vi "rsscope_core_global.vi"() -> ()   [LabVIEW 2014] (continued)
Models"="", "Instrument Options"="", "Flags"=0, "Help"="Sets the timeout between packets in a UART data stream. A new packet starts with the first start bit after the timeout.\n\nAvailable Repeated Capabilities:\nSerialBus: SB1, SB2, SB3, SB4\r\n\nRemote-control command(s):\nBUS<m>:UART:TOUT"}, {"Level"=3, "Class Only"=FALSE, "Identifier"="RSSCOPE_ATTR_PROTOCOL_UART_END_OF_FRAME", "Descriptive Name"="Protocol UART End Of Frame", "Data Type"=0, "Command"="BUS{SerialBus}:UART:EWOR", "Access"=2, "Range Table"="", "Read Callback"="", "Write Callback"="", "Supported Models"="", "Instrument Options"="", "Flags"=0, "Help"="Sets the end pattern of the packets. A new packet starts with the first start bit after the defined end pattern. This property using hexadecimal format (prefix #H).\n\nAvailable Repeated Capabilities:\nSerialBus: SB1, SB2, SB3, SB4\r\n\nRemote-control command(s):\nBUS<m>:UART:EWORd"}, {"Level"=3, "Class Only"=TRUE, "Identifier"="", "Descriptive Name"="RX", "Data Type"=0, "Command"="", "Access"=0, "Range Table"="", "Read Callback"="", "Write Callback"="", "Supported Models"="", "Instrument Options"="", "Flags"=0, "Help"="Configures UART RX properties."}, {"Level"=4, "Class Only"=FALSE, "Identifier"="RSSCOPE_ATTR_PROTOCOL_UART_RX_SOURCE", "Descriptive Name"="Protocol UART RX Source", "Data Type"=0, "Command"="BUS{SerialBus}:UART:RX:SOUR", "Access"=2, "Range Table"="rsscope_rngProtocolWaveformSource", "Read Callback"="", "Write Callback"="", "Supported Models"="", "Instrument Options"="", "Flags"=0, "Help"="Selects the input channel for the receiver signal.\n\nAvailable Repeated Capabilities:\nSerialBus: SB1, SB2, SB3, SB4\r\n\nRemote-control command(s):\nBUS<m>:UART:RX:SOURce"}, {"Level"=4, "Class Only"=FALSE, "Identifier"="RSSCOPE_ATTR_PROTOCOL_UART_RX_THRESHOLD", "Descriptive Name"="Protocol UART RX Threshold", "Data Type"=1, "Command"="BUS{SerialBus}:UART:RX:THR", "Access"=2, "Range Table"="rsscope_rngProtocolThresholdUART", "Read Callback"="", "Write Callback"="", "Supported Models"="", "Instrument Options"="", "Flags"=0, "Help"="Sets a user-defined threshold value for the Rx line.\n\nAvailable Repeated Capabilities:\nSerialBus: SB1, SB2, SB3, SB4\r\n\nRemote-control command(s):\nBUS<m>:UART:RX:THReshold"}, {"Level"=3, "Class Only"=TRUE, "Identifier"="", "Descriptive Name"="TX", "Data Type"=0, "Command"="", "Access"=0, "Range Table"="", "Read Callback"="", "Write Callback"="", "Supported Models"="", "Instrument Options"="", "Flags"=0, "Help"="Configures UART TX properties."}, {"Level"=4, "Class Only"=FALSE, "Identifier"="RSSCOPE_ATTR_PROTOCOL_UART_TX_SOURCE", "Descriptive Name"="Protocol UART TX Source", "Data Type"=0, "Command"="BUS{SerialBus}:UART:TX:SOUR", "Access"=2, "Range Table"="rsscope_rngProtocolWaveformSource", "Read Callback"="", "Write Callback"="", "Supported Models"="", "Instrument Options"="", "Flags"=0, "Help"="Selects the input channel for the transmitter signal.\n\nAvailable Repeated Capabilities:\nSerialBus: SB1, SB2, SB3, SB4\r\n\nRemote-control command(s):\nBUS<m>:UART:TX:SOURce"}, {"Level"=4, "Class Only"=FALSE, "Identifier"="RSSCOPE_ATTR_PROTOCOL_UART_TX_THRESHOLD", "Descriptive Name"="Protocol UART TX Threshold", "Data Type"=1, "Command"="BUS{SerialBus}:UART:TX:THR", "Access"=2, "Range Table"="rsscope_rngProtocolThresholdUART", "Read Callback"="", "Write Callback"="", "Supported Models"="", "Instrument Options"="", "Flags"=0, "Help"="Sets a user-defined threshold value for the Tx line.\n\nAvailable Repeated Capabilities:\nSerialBus: SB1, SB2, SB3, SB4\r\n\nRemote-control command(s):\nBUS<m>:UART:TX:THReshold"}, {"Level"=2, "Class Only"=TRUE, "Identifier"="", "Descriptive Name"="LIN", "Data Type"=0, "Command"="", "Access"=0, "Range Table"="", "Read Callback"="", "Write Callback"="", "Supported Models"="", "Instrument Options"="", "Flags"=0, "Help"="This class contains attributes that configure the LIN (Local Interconnect Network)\n\nAttributes in this class require option R&S RTO-K3."}, {"Level"=3, "Class Only"=FALSE, "Identifier"="RSSCOPE_ATTR_PROTOCOL_LIN_SOURCE", "Descriptive Name"="Protocol LIN Source", "Data Type"=0, "Command"="BUS{SerialBus}:LIN:DATA:SOUR", "Access"=2, "Range Table"="rsscope_rngProtocolWaveformSource", "Read Callback"="", "Write Callback"="", "Supported Models"="", "Instrument Options"="K0|K3", "Flags"=0, "Help"="Selects source waveform of the data line.\n\nAvailable Repeated Capabilities:\nSerialBus: SB1, SB2, SB3, SB4\r\n\nRemote-control command(s):\nBUS<m>:LIN:DATA:SOURce"}, {"Level"=3, "Class Only"=FALSE, "Identifier"="RSSCOPE_ATTR_PROTOCOL_LIN_THRESHOLD", "Descriptive Name"="Protocol LIN Threshold", "Data Type"=1, "Command"="BUS{SerialBus}:LIN:DATA:THR", "Access"=2, "Range Table"="rsscope_rngProtocolThreshold", "Read Callback"="", "Write Callback"="", "Supported Models"="", "Instrument Options"="K0|K3", "Flags"=0, "Help"="Sets threshold value for digitization of analog signals.\n\nAlternatively, you can set the threshold according to the signal technology with RSSCOPE_ATTR_PROTOCOL_LIN_TECHNOLOGY\n\nAvailable Repeated Capabilities:\nSerialBus: SB1, SB2, SB3, SB4\r\n\nRemote-control command(s):\nBUS<m>:LIN:DATA:THReshold"}, {"Level"=3, "Class Only"=FALSE, "Identifier"="RSSCOPE_ATTR_PROTOCOL_LIN_TECHNOLOGY", "Descriptive Name"="Protocol LIN Technology", "Data Type"=0, "Command"="BUS{SerialBus}:LIN:TECH", "Access"=2, "Range Table"="rsscope_rngProtocolLINTechnology", "Read Callback"="", "Write Callback"="", "Supported Models"="", "Instrument Options"="K0|K3", "Flags"=0, "Help"="Selecs the threshold voltage for various signal technologies from a list.\n\nFor user defined values set to manual and use RSSCOPE_ATTR_PROTOCOL_LIN_THRESHOLD.\n\nAvailable Repeated Capabilities:\nSerialBus: SB1, SB2, SB3, SB4\r\n\nRemote-control command(s):\nBUS<m>:LIN:TECHnology"}, {"Level"=3, "Class Only"=FALSE, "Identifier"="RSSCOPE_ATTR_PROTOCOL_LIN_STANDARD", "Descriptive Name"="Protocol LIN Standard", "Data Type"=0, "Command"="BUS{SerialBus}:LIN:STAN", "Access"=2, "Range Table"="rsscope_rngProtocolLINStandard", "Read Callback"="", "Write Callback"="", "Supported Models"="", "Instrument Options"="K0|K3", "Flags"=0, "Help"="This attribute selects the version of the LIN standard.\n\nAvailable Repeated Capabilities:\nSerialBus: SB1, SB2, SB3, SB4\r\n\nRemote-control command(s):\nBUS<m>:LIN:STANdard"}, {"Level"=3, "Class Only"=FALSE, "Identifier"="RSSCOPE_ATTR_PROTOCOL_LIN_BIT_RATE", "Descriptive Name"="Protocol LIN Bit Rate", "Data Type"=0, "Command"="BUS{SerialBus}:LIN:BITR", "Access"=2, "Range Table"="rsscope_rngProtocolLINBitRate", "Read Callback"="", "Write Callback"="", "Supported Models"="", "Instrument Options"="K0|K3", "Flags"=0, "Help"="Sets the number of transmitted bits per second.\n\nNote(s):\n(1) For LIN standard &apos;J2602&apos;, the bit rate is 10417 kbit/s and cannot be changed.\n\nAvailable Repeated Capabilities:\nSerialBus: SB1, SB2, SB3, SB4\r\n\nRemote-control command(s):\nBUS<m>:LIN:BITRate"}, {"Level"=3, "Class Only"=FALSE, "Identifier"="RSSCOPE_ATTR_PROTOCOL_LIN_POLARITY", "Descriptive Name"="Protocol LIN Polarity", "Data Type"=0, "Command"="BUS{SerialBus}:LIN:POL", "Access"=2, "Range Table"="rsscope_rngProtocolPolarity", "Read Callback"="", "Write Callback"="", "Supported Models"="", "Instrument Options"="K0|K3", "Flags"=0, "Help"="Sets the idle state of the bus. The idle state is the rezessive state and corresponds to a logic 1.\n\nAvailable Repeated Capabilities:\nSerialBus: SB1, SB2, SB3, SB4\r\n\nRemote-control command(s):\nBUS<m>:LIN:POLarity"}, {"Level"=3, "Class Only"=FALSE, "Identifier"="RSSCOPE_ATTR_PROTOCOL_LIN_SELECTED_FRAME", "Descriptive Name"="Protocol LIN Selected Frame", "Data Type"=0, "Command"="", "Access"=2, "Range Table"="", "Read Callback"="", "Write Callback"="", "Supported Models"="", "Instrument Options"="", "Flags"=0, "Help"="Sets selector repeated capability Frame.\n\nAvailable Repeated Capabilities:\nNone\n\nRemote-control command(s):\ncmd"}, {"Level"=3, "Class Only"=FALSE, "Identifier"="RSSCOPE_ATTR_PROTOCOL_LIN_FRAME_COUNT", "Descriptive Name"="Protocol LIN Frame Count", "Data Type"=0, "Command"="BUS{SerialBus}:LIN:FCO?", "Access"=0, "Range Table"="", "Read Callback"="", "Write Callback"="", "Supported Models"="", "Instrument Options"="K0|K3", "Flags"=0, "Help"="Returns number of decoded frames.\n\nAvailable Repeated Capabilities:\nSerialBus: SB1, SB2, SB3, SB4\r\n\nRemote-control command(s):\nBUS<m>:LIN:FCOunt?"}, {"Level"=3, "Class Only"=FALSE, "Identifier"="RSSCOPE_ATTR_PROTOCOL_LIN_FRAME_STATUS", "Descriptive Name"="Protocol LIN Frame Status", "Data Type"=0, "Command"="BUS{SerialBus}:LIN:FRAM<Frame>:STAT?", "Access"=0, "Range Table"="RsScope_rngLINFrameStatus", "Read Callback"="rsscope_FormatLINFrameRepCapInt32_ReadCallback.vi", "Write Callback"="", "Supported Models"="", "Instrument Options"="K3", "Flags"=0, "Help"="The overall state of the frame.\n\nAvailable Repeated Capabilities:\nSerialBus: SB1, SB2, SB3, SB4\r\n\nRemote-control command(s):\nBUS<m>:LIN:FRAMe<n>:STATus?"}, {"Level"=3, "Class Only"=FALSE, "Identifier"="RSSCOPE_ATTR_PROTOCOL_LIN_FRAME_START", "Descriptive Name"="Protocol LIN Frame Start", "Data Type"=1, "Command"="BUS{SerialBus}:LIN:FRAM<Frame>:STAR?", "Access"=0, "Range Table"="", "Read Callback"="rsscope_FormatLINFrameRepCapReal64_ReadCallback.vi", "Write Callback"="", "Supported Models"="", "Instrument Options"="K3", "Flags"=0, "Help"="Return the start time of the selected frame.\n\nAvailable Repeated Capabilities:\nSerialBus: SB1, SB2, SB3, SB4\r\n\nRemote-control command(s):\nBUS<m>:LIN:FRAMe<n>:STARt?"}, {"Level"=3, "Class Only"=FALSE, "Identifier"="RSSCOPE_ATTR_PROTOCOL_LIN_FRAME_STOP", "Descriptive Name"="Protocol LIN Frame Stop", "Data Type"=1, "Command"="BUS{SerialBus}:LIN:FRAM<Frame>:STOP?", "Access"=0, "Range Table"="", "Read Callback"="rsscope_FormatLINFrameRepCapReal64_ReadCallback.vi", "Write Callback"="", "Supported Models"="", "Instrument Options"="K3", "Flags"=0, "Help"="Return the stop time of the selected frame.\n\nAvailable Repeated Capabilities:\nSerialBus: SB1, SB2, SB3, SB4\r\n\nRemote-control command(s):\nBUS<m>:LIN:FRAMe<n>:STOP?"}, {"Level"=3, "Class Only"=FALSE, "Identifier"="RSSCOPE_ATTR_PROTOCOL_LIN_FRAME_VERSION", "Descriptive Name"="Protocol LIN Frame Version", "Data Type"=0, "Command"="BUS{SerialBus}:LIN:FRAM<Frame>:VERS?", "Access"=0, "Range Table"="RsScope_rngLINFrameVersion", "Read Callback"="rsscope_FormatLINFrameRepCapInt32_ReadCallback.vi", "Write Callback"="", "Supported Models"="", "Instrument Options"="K3", "Flags"=0, "Help"="Returns the version of the LIN standard for the specified frame.\n\nAvailable Repeated Capabilities:\nSerialBus: SB1, SB2, SB3, SB4\r\n\nRemote-control command(s):\nBUS<m>:LIN:FRAMe<n>:VERSion?"}, {"Level"=3, "Class Only"=FALSE, "Identifier"="RSSCOPE_ATTR_PROTOCOL_LIN_FRAME_ID_VALUE", "Descriptive Name"="Protocol LIN Frame ID Value", "Data Type"=0, "Command"="BUS{SerialBus}:LIN:FRAM<Frame>:IDV?", "Access"=0, "Range Table"="", "Read Callback"="rsscope_FormatLINFrameRepCapInt32_ReadCallback.vi", "Write Callback"="", "Supported Models"="", "Instrument Options"="K3", "Flags"=0, "Help"="Returns the version of the LIN standard for the specified frame.\n\nAvailable Repeated Capabilities:\nSerialBus: SB1, SB2, SB3, SB4\r\n\nRemote-control command(s):\nBUS<m>:LIN:FRAMe<n>:IDValue?"}, {"Level"=3, "Class Only"=FALSE, "Identifier"="RSSCOPE_ATTR_PROTOCOL_LIN_FRAME_ID_PARITY", "Descriptive Name"="Protocol LIN Frame ID Parity", "Data Type"=0, "Command"="BUS{SerialBus}:LIN:FRAM<Frame>:IDPV?", "Access"=0, "Range Table"="", "Read Callback"="rsscope_FormatLINFrameRepCapInt32_ReadCallback.vi", "Write Callback"="", "Supported Models"="", "Instrument Options"="K3", "Flags"=0, "Help"="Returns the value of the identifier parity bits of the selected frame.\n\nAvailable Repeated Capabilities:\nSerialBus: SB1, SB2, SB3, SB4\r\n\nRemote-control command(s):\nBUS<m>:LIN:FRAMe<n>:IDPValue?"}, {"Level"=3, "Class Only"=FALSE, "Identifier"="RSSCOPE_ATTR_PROTOCOL_LIN_FRAME_ID_STATUS", "Descriptive Name"="Protocol LIN Frame ID Status", "Data Type"=0, "Command"="BUS{SerialBus}:LIN:FRAM<Frame>:IDST?", "Access"=0, "Range Table"="RsScope_rngLINFieldStatus", "Read Callback"="rsscope_FormatLINFrameRepCapInt32_ReadCallback.vi", "Write Callback"="", "Supported Models"="", "Instrument Options"="K3", "Flags"=0, "Help"="Returns the identifier state of the selected frame.\n\nAvailable Repeated Capabilities:\nSerialBus: SB1, SB2, SB3, SB4\r\n\nRemote-control command(s):\nBUS<m>:LIN:FRAMe<n>:IDSTate?"}, {"Level"=3, "Class Only"=FALSE, "Identifier"="RSSCOPE_ATTR_PROTOCOL_LIN_FRAME_SYNC_STATUS", "Descriptive Name"="Protocol LIN Frame Sync Status", "Data Type"=0, "Command"="BUS{SerialBus}:LIN:FRAM<Frame>:SYST?", "Access"=0, "Range Table"="RsScope_rngLINFieldStatus", "Read Callback"="rsscope_FormatLINFrameRepCapInt32_ReadCallback.vi", "Write Callback"="", "Supported Models"="", "Instrument Options"="K3", "Flags"=0, "Help"="Returns the state of the sync field for the specified frame.\n\nAvailable Repeated Capabilities:\nSerialBus: SB1, SB2, SB3, SB4\r\n\nRemote-control command(s):\nBUS<m>:LIN:FRAMe<n>:SYSTate?"}, {"Level"=3, "Class Only"=FALSE, "Identifier"="RSSCOPE_ATTR_PROTOCOL_LIN_FRAME_CHECKSUM_STATUS", "Descriptive Name"="Protocol LIN Frame Checksum Status", "Data Type"=0, "Command"="BUS{SerialBus}:LIN:FRAM<Frame>:CSST?", "Access"=0, "Range Table"="RsScope_rngLINFieldStatus", "Read Callback"="rsscope_FormatLINFrameRepCapInt32_ReadCallback.vi", "Write Callback"="", "Supported Models"="", "Instrument Options"="K3", "Flags"=0, "Help"="Returns the checksum state of the specified frame.\n\nAvailable Repeated Capabilities:\nSerialBus: SB1, SB2, SB3, SB4\r\n\nRemote-control command(s):\nBUS<m>:LIN:FRAMe<n>:CSSTate?"}, {"Level"=3, "Class Only"=FALSE, "Identifier"="RSSCOPE_ATTR_PROTOCOL_LIN_FRAME_CHECKSUM_VALUE", "Descriptive Name"="Protocol LIN Frame Checksum Value", "Data Type"=0, "Command"="BUS{SerialBus}:LIN:FRAM<Frame>:CSV?", "Access"=0, "Range Table"="", "Read Callback"="rsscope_FormatLINFrameRepCapInt32_ReadCallback.vi", "Write Callback"="", "Supported Models"="", "Instrument Options"="K3", "Flags"=0, "Help"="Returns the checksum value of the specified frame.\n\nAvailable Repeated Capabilities:\nSerialBus: SB1, SB2, SB3, SB4\r\n\nRemote-control command(s):\nBUS<m>:LIN:FRAMe<n>:CSValue?"}, {"Level"=3, "Class Only"=FALSE, "Identifier"="RSSCOPE_ATTR_PROTOCOL_LIN_FRAME_BIT_RATE", "Descriptive Name"="Protocol LIN Frame Bit Rate", "Data Type"=5, "Command"="BUS{SerialBus}:LIN:FRAM<Frame>:BITR?", "Access"=0, "Range Table"="", "Read Callback"="rsscope_FormatLINFrameRepCapInt64_ReadCallback.vi", "Write Callback"="", "Supported Models"="", "Instrument Options"="K3", "Flags"=0, "Help"="Returns the primary bit rate.\n\nAvailable Repeated Capabilities:\nSerialBus: SB1, SB2, SB3, SB4\r\n\nRemote-control command(s):\nBUS<m>:LIN:FRAMe<n>:BITRate?"}, {"Level"=3, "Class Only"=FALSE, "Identifier"="RSSCOPE_ATTR_PROTOCOL_LIN_FRAME_LABEL", "Descriptive Name"="Protocol LIN Frame Label", "Data Type"=2, "Command"="BUS{SerialBus}:LIN:FRAM<Frame>:SYMB?", "Access"=0, "Range Table"="", "Read Callback"="rsscope_FormatLINFrameRepCapString_ReadCallback.vi", "Write Callback"="", "Supported Models"="", "Instrument Options"="K3", "Flags"=0, "Help"="This attribute returns the symbolic label of the specified frame if the label list is enabled.\n\nAvailable Repeated Capabilities:\nSerialBus: SB1, SB2, SB3, SB4\r\n\nRemote-control command(s):\nBUS<m>:LIN:FRAMe<n>:SYMBol?"}, {"Level"=3, "Class Only"=FALSE, "Identifier"="RSSCOPE_ATTR_PROTOCOL_LIN_SELECTED_BYTE", "Descriptive Name"="Protocol LIN Selected Byte", "Data Type"=0, "Command"="", "Access"=2, "Range Table"="", "Read Callback"="", "Write Callback"="", "Supported Models"="", "Instrument Options"="", "Flags"=0, "Help"="Sets selector repeated capability Byte.\n\nAvailable Repeated Capabilities:\nNone\n\nRemote-control command(s):\ncmd"}, {"Level"=3, "Class Only"=FALSE, "Identifier"="RSSCOPE_ATTR_PROTOCOL_LIN_FRAME_BYTE_DATA", "Descriptive Name"="Protocol LIN Frame Byte Data", "Data Type"=0, "Command"="BUS{SerialBus}:LIN:FRAM<Frame>:BYTE<Byte>:VAL?", "Access"=0, "Range Table"="", "Read Callback"="rsscope_FormatLINByteRepCapInt32_ReadCallback.vi", "Write Callback"="", "Supported Models"="", "Instrument Options"="K3", "Flags"=0, "Help"="Value of the specified byte.\n\nAvailable Repeated Capabilities:\nSerialBus: SB1, SB2, SB3, SB4\r\n\nRemote-control command(s):\nBUS<m>:LIN:FRAMe<n>:BYTE<o>:VALue?"}, {"Level"=3, "Class Only"=FALSE, "Identifier"="RSSCOPE_ATTR_PROTOCOL_LIN_FRAME_BYTE_STATUS", "Descriptive Name"="Protocol LIN Frame Byte Status", "Data Type"=0, "Command"="BUS{SerialBus}:LIN:FRAM<Frame>:BYTE<Byte>:STAT?", "Access"=0, "Range Table"="RsScope_rngLINFieldStatus", "Read Callback"="rsscope_FormatLINByteRepCapInt32_ReadCallback.vi", "Write Callback"="", "Supported Models"="", "Instrument Options"="K3", "Flags"=0, "Help"="Returns the data state for the specified frame.\n\nAvailable Repeated Capabilities:\nSerialBus: SB1, SB2, SB3, SB4\r\n\nRemote-control command(s):\nBUS<m>:LIN:FRAMe<n>:BYTE<o>:STATe?"}, {"Level"=2, "Class Only"=TRUE, "Identifier"="", "Descriptive Name"="CAN", "Data Type"=0, "Command"="", "Access"=0, "Range Table"="", "Read Callback"="", "Write Callback"="", "Supported Models"="", "Instrument Options"="", "Flags"=0, "Help"="This class contains attributes that configure the CAN (Controller Area Network)\n\nAttributes in this class require option R&S RTO-K3."}, {"Level"=3, "Class Only"=FALSE, "Identifier"="RSSCOPE_ATTR_PROTOCOL_CAN_SOURCE", "Descriptive Name"="Protocol CAN Source", "Data Type"=0, "Command"="BUS{SerialBus}:CAN:DATA:SOUR", "Access"=2, "Range Table"="rsscope_rngProtocolWaveformSource", "Read Callback"="", "Write Callback"="", "Supported Models"="", "Instrument Options"="K0|K3", "Flags"=0, "Help"="Selects source waveform of the data line.\n\nAvailable Repeated Capabilities:\nSerialBus: SB1, SB2, SB3, SB4\r\n\nRemote-control command(s):\nBUS<m>:CAN:DATA:SOURce"}, {"Level"=3, "Class Only"=FALSE, "Identifier"="RSSCOPE_ATTR_PROTOCOL_CAN_LINE_TYPE", "Descriptive Name"="Protocol CAN Line Type", "Data Type"=0, "Command"="BUS{SerialBus}:CAN:TYPE", "Access"=2, "Range Table"="rsscope_rngProtocolCANLineType", "Read Callback"="", "Write Callback"="", "Supported Models"="", "Instrument Options"="K0|K3", "Flags"=0, "Help"="Selects the CAN-High or CAN-Low line. Both lines are required for differential signal transmission used by CAN.\n\nAvailable Repeated Capabilities:\nSerialBus: SB1, SB2, SB3, SB4\r\n\nRemote-control command(s):\nBUS<m>:CAN:TYPE"}, {"Level"=3, "Class Only"=FALSE, "Identifier"="RSSCOPE_ATTR_PROTOCOL_CAN_THRESHOLD", "Descriptive Name"="Protocol CAN Threshold", "Data Type"=1, "Command"="BUS{SerialBus}:CAN:DATA:THR", "Access"=2, "Range Table"="rsscope_rngProtocolThreshold", "Read Callback"="", "Write Callback"="", "Supported Models"="", "Instrument Options"="K0|K3", "Flags"=0, "Help"="Sets threshold value for digitization of analog signals.\n\nAlternatively, you can set the threshold according to the signal technology with RSSCOPE_ATTR_PROTOCOL_CAN_TECHNOLOGY\n\nAvailable Repeated Capabilities:\nSerialBus: SB1, SB2, SB3, SB4\r\n\nRemote-control command(s):\nBUS<m>:CAN:DATA:THReshold"}, {"Level"=3, "Class Only"=FALSE, "Identifier"="RSSCOPE_ATTR_PROTOCOL_CAN_TECHNOLOGY", "Descriptive Name"="Protocol CAN Technology", "Data Type"=0, "Command"="BUS{SerialBus}:CAN:TECH", "Access"=2, "Range Table"="rsscope_rngProtocolCANTechnology", "Read Callback"="", "Write Callback"="", "Supported Models"="", "Instrument Options"="K0|K3", "Flags"=0, "Help"="Selecs the threshold voltage for various signal technologies from a list.\n\nFor user defined values set to manual and use RSSCOPE_ATTR_PROTOCOL_LIN_THRESHOLD.\n\nAvailable Repeated Capabilities:\nSerialBus: SB1, SB2, SB3, SB4\r\n\nRemote-control command(s):\nBUS<m>:CAN:TECHnology"}, {"Level"=3, "Class Only"=FALSE, "Identifier"="RSSCOPE_ATTR_PROTOCOL_CAN_BIT_RATE", "Descriptive Name"="Protocol CAN Bit Rate", "Data Type"=0, "Command"="BUS{SerialBus}:CAN:BITR", "Access"=2, "Range Table"="rsscope_rngProtocolCANBitRate", "Read Callback"="", "Write Callback"="", "Supported Models"="", "Instrument Options"="K0|K3", "Flags"=0, "Help"="Sets the number of transmitted bits per second.\n\nAvailable Repeated Capabilities:\nSerialBus: SB1, SB2, SB3, SB4\r\n\nRemote-control command(s):\nBUS<m>:CAN:BITRate"}, {"Level"=3, "Class Only"=FALSE, "Identifier"="RSSCOPE_ATTR_PROTOCOL_CAN_FD_ENABLED", "Descriptive Name"="Protocol CAN FD Enabled", "Data Type"=3, "Command"="BUS{SerialBus}:CAN:FDAT:ENAB", "Access"=2, "Range Table"="", "Read Callback"="", "Write Callback"="", "Supported Models"="", "Instrument Options"="K9", "Flags"=0, "Help"="Enables the CAN FD protocol configuration.\n\nAvailable Repeated Capabilities:\nSerialBus: SB1, SB2, SB3, SB4\r\n\nRemote-control command(s):\nBUS<m>:CAN:FDATa:ENABle"}, {"Level"=3, "Class Only"=FALSE, "Identifier"="RSSCOPE_ATTR_PROTOCOL_CAN_FD_BIT_RATE", "Descriptive Name"="Protocol CAN FD Bit Rate", "Data Type"=0, "Command"="BUS{SerialBus}:CAN:FDAT:DBIT", "Access"=2, "Range Table"="rsscope_rngProtocolCANFDBitRate", "Read Callback"="", "Write Callback"="", "Supported Models"="", "Instrument Options"="K9", "Flags"=0, "Help"="Sets the bit rate of the data phase. The data rate can be higher than the arbitration rate, but it is uniform and fixed for a given CAN FD bus.\n\nAvailable Repeated Capabilities:\nSerialBus: SB1, SB2, SB3, SB4\r\n\nRemote-control command(s):\nBUS<m>:CAN:FDATa:DBITrate"}, {"Level"=3, "Class Only"=FALSE, "Identifier"="RSSCOPE_ATTR_PROTOCOL_CAN_JUMP_WIDTH", "Descriptive Name"="Protocol CAN Jump Width", "Data Type"=1, "Command"="BUS{SerialBus}:CAN:JWID", "Access"=2, "Range Table"="rsscope_rngProtocolCANJumpWidth", "Read Callback"="", "Write Callback"="", "Supported Models"="", "Instrument Options"="K0|K3", "Flags"=0, "Help"="This attribute configures maximum number of time quanta for phase correction. This mean Time segment1 may be lengthened or Time segment2 may be shortened due to resynchronization.\n\nAvailable Repeated Capabilities:\nSerialBus: SB1, SB2, SB3, SB4\r\n\nRemote-control command(s):\nBUS<m>:CAN:JWIDth"}, {"Level"=3, "Class Only"=FALSE, "Identifier"="RSSCOPE_ATTR_PROTOCOL_CAN_SAMPLE_POINT_REL", "Descriptive Name"="Protocol CAN Sample Point Rel", "Data Type"=1, "Command"="BUS{SerialBus}:CAN:SAMP", "Access"=2, "Range Table"="rsscope_rngProtocolCANSamplePoint", "Read Callback"="", "Write Callback"="", "Supported Models"="", "Instrument Options"="K0|K3", "Flags"=0, "Help"="Sets the position of the sample point within the bit in percent ot the nominal bit time.\n\nAvailable Repeated Capabilities:\nSerialBus: SB1, SB2, SB3, SB4\r\n\nRemote-control command(s):\nBUS<m>:CAN:SAMPlepoint"}, {"Level"=3, "Class Only"=FALSE, "Identifier"="RSSCOPE_ATTR_PROTOCOL_CAN_FD_JUMP_WIDTH", "Descriptive Name"="Protocol CAN FD Jump Width", "Data Type"=1, "Command"="BUS{SerialBus}:CAN:FDAT:JWID", "Access"=2, "Range Table"="rsscope_rngProtocolCANJumpWidth", "Read Callback"="", "Write Callback"="", "Supported Models"="", "Instrument Options"="K0|K3", "Flags"=0, "Help"="This attribute configures maximum number of time quanta for phase correction. This mean Time segment1 may be lengthened or Time segment2 may be shortened due to resynchronization.\n\nAvailable Repeated Capabilities:\nSerialBus: SB1, SB2, SB3, SB4\r\n\nRemote-control command(s):\nBUS<m>:CAN:FDATa:JWIDth"}, {"Level"=3, "Class Only"=FALSE, "Identifier"="RSSCOPE_ATTR_PROTOCOL_CAN_FD_SAMPLE_POINT_REL", "Descriptive Name"="Protocol CAN FD Sample Point Rel", "Data Type"=1, "Command"="BUS{SerialBus}:CAN:FDAT:SAMP", "Access"=2, "Range Table"="rsscope_rngProtocolCANSamplePoint", "Read Callback"="", "Write Callback"="", "Supported Models"="", "Instrument Options"="K0|K3", "Flags"=0, "Help"="Sets the position of the sample point within the bit in percent ot the nominal bit time.\n\nAvailable Repeated Capabilities:\nSerialBus: SB1, SB2, SB3, SB4\r\n\nRemote-control command(s):\nBUS<m>:CAN:FDATa:SAMPlepoint"}, {"Level"=3, "Class Only"=FALSE, "Identifier"="RSSCOPE_ATTR_PROTOCOL_CAN_FD_STANDARD", "Descriptive Name"="Protocol CAN FD Standard", "Data Type"=0, "Command"="BUS{SerialBus}:CAN:FDAT:PST", "Access"=2, "Range Table"="RsScope_rngCANFDStandard", "Read Callback"="", "Write Callback"="", "Supported Models"="", "Instrument Options"="K3", "Flags"=0, "Help"="Only available for CAN FD buses. Selects whether the tested signal is an ISO CAN FD signal or not.\n\nAvailable Repeated Capabilities:\nSerialBus: SB1, SB2, SB3, SB4\r\n\nRemote-control command(s):\nBUS<m>:CAN:FDATa:PSTandard"}, {"Level"=3, "Class Only"=FALSE, "Identifier"="RSSCOPE_ATTR_PROTOCOL_CAN_SELECTED_FRAME", "Descriptive Name"="Protocol CAN Selected Frame", "Data Type"=0, "Command"="", "Access"=2, "Range Table"="", "Read Callback"="", "Write Callback"="", "Supported Models"="", "Instrument Options"="", "Flags"=0, "Help"="Sets selector repeated capability Frame.\n\nAvailable Repeated Capabilities:\nNone\n\nRemote-control command(s):\ncmd"}, {"Level"=3, "Class Only"=FALSE, "Identifier"="RSSCOPE_ATTR_PROTOCOL_CAN_FRAME_COUNT", "Descriptive Name"="Protocol CAN Frame Count", "Data Type"=0, "Command"="BUS{SerialBus}:CAN:FCO?", "Access"=0, "Range Table"="", "Read Callback"="", "Write Callback"="", "Supported Models"="", "Instrument Options"="K0|K3", "Flags"=0, "Help"="Returns number of decoded frames.\n\nAvailable Repeated Capabilities:\nSerialBus: SB1, SB2, SB3, SB4\r\n\nRemote-control command(s):\nBUS<m>:CAN:FCOunt?"}, {"Level"=3, "Class Only"=FALSE, "Identifier"="RSSCOPE_ATTR_PROTOCOL_CAN_FRAME_STANDARD", "Descriptive Name"="Protocol CAN Frame Standard", "Data Type"=0, "Command"="BUS{SerialBus}:CAN:FDAT:FRAM<Frame>:STAN?", "Access"=0, "Range Table"="rsscope_rngCANStandard", "Read Callback"="rsscope_FormatCANFrameRepCapInt32_ReadCallback.vi", "Write Callback"="", "Supported Models"="", "Instrument Options"="K9", "Flags"=0, "Help"="Returns the CAN standard.\n\nAvailable Repeated Capabilities:\nSerialBus: SB1, SB2, SB3, SB4\r\n\nRemote-control command(s):\nBUS<m>:CAN:FDATa:FRAMe<n>:STANdard?"}, {"Level"=3, "Class Only"=FALSE, "Identifier"="RSSCOPE_ATTR_PROTOCOL_CAN_FRAME_STATUS", "Descriptive Name"="Protocol CAN Frame Status", "Data Type"=0, "Command"="BUS{SerialBus}:CAN:FRAM<Frame>:STAT?", "Access"=0, "Range Table"="RsScope_rngCANFrameStatus", "Read Callback"="rsscope_FormatCANFrameRepCapInt32_ReadCallback.vi", "Write Callback"="", "Supported Models"="", "Instrument Options"="K3", "Flags"=0, "Help"="The overall state of the frame.\n\nAvailable Repeated Capabilities:\nSerialBus: SB1, SB2, SB3, SB4\r\n\nRemote-control command(s):\nBUS<m>:CAN:FRAMe<n>:STATus?"}, {"Level"=3, "Class Only"=FALSE, "Identifier"="RSSCOPE_ATTR_PROTOCOL_CAN_FRAME_START", "Descriptive Name"="Protocol CAN Frame Start", "Data Type"=1, "Command"="BUS{SerialBus}:CAN:FRAM<Frame>:STAR?", "Access"=0, "Range Table"="", "Read Callback"="rsscope_FormatCANFrameRepCapReal64_ReadCallback.vi", "Write Callback"="", "Supported Models"="", "Instrument Options"="K3", "Flags"=0, "Help"="Return the start time of the selected frame.\n\nAvailable Repeated Capabilities:\nSerialBus: SB1, SB2, SB3, SB4\r\n\nRemote-control command(s):\nBUS<m>:CAN:FRAMe<n>:STARt?"}, {"Level"=3, "Class Only"=FALSE, "Identifier"="RSSCOPE_ATTR_PROTOCOL_CAN_FRAME_STOP", "Descriptive Name"="Protocol CAN Frame Stop", "Data Type"=1, "Command"="BUS{SerialBus}:CAN:FRAM<Frame>:STOP?", "Access"=0, "Range Table"="", "Read Callback"="rsscope_FormatCANFrameRepCapReal64_ReadCallback.vi", "Write Callback"="", "Supported Models"="", "Instrument Options"="K3", "Flags"=0, "Help"="Return the stop time of the selected frame.\n\nAvailable Repeated Capabilities:\nSerialBus: SB1, SB2, SB3, SB4\r\n\nRemote-control command(s):\nBUS<m>:CAN:FRAMe<n>:STOP?"}, {"Level"=3, "Class Only"=FALSE, "Identifier"="RSSCOPE_ATTR_PROTOCOL_CAN_FRAME_TYPE", "Descriptive Name"="Protocol CAN Frame Type", "Data Type"=0, "Command"="BUS{SerialBus}:CAN:FRAM<Frame>:TYPE?", "Access"=0, "Range Table"="RsScope_rngProtocolCANFrameType", "Read Callback"="rsscope_FormatCANFrameRepCapInt32_ReadCallback.vi", "Write Callback"="", "Supported Models"="", "Instrument Options"="K3", "Flags"=0, "Help"="Returns the frame type of the selected frame.\n\nAvailable Repeated Capabilities:\nSerialBus: SB1, SB2, SB3, SB4\r\n\nRemote-control command(s):\nBUS<m>:CAN:FRAMe<n>:TYPE?"}, {"Level"=3, "Class Only"=FALSE, "Identifier"="RSSCOPE_ATTR_PROTOCOL_CAN_FRAME_ID_TYPE", "Descriptive Name"="Protocol CAN Frame ID Type", "Data Type"=0, "Command"="BUS{SerialBus}:CAN:FRAM<Frame>:IDTY?", "Access"=0, "Range Table"="RsScope_rngCANFrameIDType", "Read Callback"="rsscope_FormatCANFrameRepCapInt32_ReadCallback.vi", "Write Callback"="", "Supported Models"="", "Instrument Options"="K3", "Flags"=0, "Help"="Returns the identifier type of the selected frame, the identifier format of data and remote frames.\n\nAvailable Repeated Capabilities:\nSerialBus: SB1, SB2, SB3, SB4\r\n\nRemote-control command(s):\nBUS<m>:CAN:FRAMe<n>:IDTYpe?"}, {"Level"=3, "Class Only"=FALSE, "Identifier"="RSSCOPE_ATTR_PROTOCOL_CAN_FRAME_ID_VALUE", "Descriptive Name"="Protocol CAN Frame ID Value", "Data Type"=0, "Command"="BUS{SerialBus}:CAN:FRAM<Frame>:IDV?", "Access"=0, "Range Table"="", "Read Callback"="rsscope_FormatCANFrameRepCapInt32_ReadCallback.vi", "Write Callback"="", "Supported Models"="", "Instrument Options"="K3", "Flags"=0, "Help"="Returns the identifier value of the selected frame.\n\nAvailable Repeated Capabilities:\nSerialBus: SB1, SB2, SB3, SB4\r\n\nRemote-control command(s):\nBUS<m>:CAN:FRAMe<n>:IDValue?"}, {"Level"=3, "Class Only"=FALSE, "Identifier"="RSSCOPE_ATTR_PROTOCOL_CAN_FRAME_ID_STATUS", "Descriptive Name"="Protocol CAN Frame ID Status", "Data Type"=0, "Command"="BUS{SerialBus}:CAN:FRAM<Frame>:IDST?", "Access"=0, "Range Table"="RsScope_rngCANFrameMessageStatus", "Read Callback"="rsscope_FormatCANFrameRepCapInt32_ReadCallback.vi", "Write Callback"="", "Supported Models"="", "Instrument Options"="K3", "Flags"=0, "Help"="Return the identifier state.\n\nAvailable Repeated Capabilities:\nSerialBus: SB1, SB2, SB3, SB4\r\n\nRemote-control command(s):\nBUS<m>:CAN:FRAMe<n>:IDSTate?"}, {"Level"=3, "Class Only"=FALSE, "Identifier"="RSSCOPE_ATTR_PROTOCOL_CAN_FRAME_DLC_VALUE", "Descriptive Name"="Protocol CAN Frame DLC Value", "Data Type"=0, "Command"="BUS{SerialBus}:CAN:FRAM<Frame>:DLCV?", "Access"=0, "Range Table"="", "Read Callback"="rsscope_FormatCANFrameRepCapInt32_ReadCallback.vi", "Write Callback"="", "Supported Models"="", "Instrument Options"="K3", "Flags"=0, "Help"="Returns the field state of the selected frame.\n\nAvailable Repeated Capabilities:\nSerialBus: SB1, SB2, SB3, SB4\r\n\nRemote-control command(s):\nBUS<m>:CAN:FRAMe<n>:DLCValue?"}, {"Level"=3, "Class Only"=FALSE, "Identifier"="RSSCOPE_ATTR_PROTOCOL_CAN_FRAME_DLC_STATUS", "Descriptive Name"="Protocol CAN Frame DLC Status", "Data Type"=0, "Command"="BUS{SerialBus}:CAN:FRAM<Frame>:DLCS?", "Access"=0, "Range Table"="RsScope_rngCANFrameMessageStatus", "Read Callback"="rsscope_FormatCANFrameRepCapInt32_ReadCallback.vi", "Write Callback"="", "Supported Models"="", "Instrument Options"="K3", "Flags"=0, "Help"="Returns the field state of the selected frame.\n\nAvailable Repeated Capabilities:\nSerialBus: SB1, SB2, SB3, SB4\r\n\nRemote-control command(s):\nBUS<m>:CAN:FRAMe<n>:DLCState?"}, {"Level"=3, "Class Only"=FALSE, "Identifier"="RSSCOPE_ATTR_PROTOCOL_CAN_FRAME_ACK_VALUE", "Descriptive Name"="Protocol CAN Frame Ack Value", "Data Type"=0, "Command"="BUS{SerialBus}:CAN:FRAM<Frame>:ACKV?", "Access"=0, "Range Table"="", "Read Callback"="rsscope_FormatCANFrameRepCapInt32_ReadCallback.vi", "Write Callback"="", "Supported Models"="", "Instrument Options"="K3", "Flags"=0, "Help"="Returns the field state of the selected frame.\n\nAvailable Repeated Capabilities:\nSerialBus: SB1, SB2, SB3, SB4\r\n\nRemote-control command(s):\nBUS<m>:CAN:FRAMe<n>:ACKValue?"}, {"Level"=3, "Class Only"=FALSE, "Identifier"="RSSCOPE_ATTR_PROTOCOL_CAN_FRAME_ACK_STATUS", "Descriptive Name"="Protocol CAN Frame Ack Status", "Data Type"=0, "Command"="BUS{SerialBus}:CAN:FRAM<Frame>:ACKS?", "Access"=0, "Range Table"="RsScope_rngCANFrameMessageStatus", "Read Callback"="rsscope_FormatCANFrameRepCapInt32_ReadCallback.vi", "Write Callback"="", "Supported Models"="", "Instrument Options"="K3", "Flags"=0, "Help"="Returns the field state of the selected frame.\n\nAvailable Repeated Capabilities:\nSerialBus: SB1, SB2, SB3, SB4\r\n\nRemote-control command(s):\nBUS<m>:CAN:FRAMe<n>:ACKState?"}, {"Level"=3, "Class Only"=FALSE, "Identifier"="RSSCOPE_ATTR_PROTOCOL_CAN_FRAME_BIT_RATE", "Descriptive Name"="Protocol CAN Frame Bit Rate", "Data Type"=5, "Command"="BUS{SerialBus}:CAN:FRAM<Frame>:BITR?", "Access"=0, "Range Table"="RsScope_rngCANFrameBitRate", "Read Callback"="rsscope_FormatCANFrameRepCapInt64_ReadCallback.vi", "Write Callback"="", "Supported Models"="", "Instrument Options"="", "Flags"=0, "Help"="Returns the primary bit rate.\n\nAvailable Repeated Capabilities:\nSerialBus: SB1, SB2, SB3, SB4\r\n\nRemote-control command(s):\nBUS<m>:CAN:FRAMe<n>:BITRate?"}, {"Level"=3, "Class Only"=FALSE, "Identifier"="RSSCOPE_ATTR_PROTOCOL_CAN_FRAME_CRC_VALUE", "Descriptive Name"="Protocol CAN Frame CRC Value", "Data Type"=0, "Command"="BUS{SerialBus}:CAN:FRAM<Frame>:CSV?", "Access"=0, "Range Table"="", "Read Callback"="rsscope_FormatCANFrameRepCapInt32_ReadCallback.vi", "Write Callback"="", "Supported Models"="", "Instrument Options"="K3", "Flags"=0, "Help"="Returns the field state of the selected frame.\n\nAvailable Repeated Capabilities:\nSerialBus: SB1, SB2, SB3, SB4\r\n\nRemote-control command(s):\nBUS<m>:CAN:FRAMe<n>:CSValue?"}, {"Level"=3, "Class Only"=FALSE, "Identifier"="RSSCOPE_ATTR_PROTOCOL_CAN_FRAME_CRC_STATUS", "Descriptive Name"="Protocol CAN Frame CRC Status", "Data Type"=0, "Command"="BUS{SerialBus}:CAN:FRAM<Frame>:CSST?", "Access"=0, "Range Table"="RsScope_rngCANFrameMessageStatus", "Read Callback"="rsscope_FormatCANFrameRepCapInt32_ReadCallback.vi", "Write Callback"="", "Supported Models"="", "Instrument Options"="K3", "Flags"=0, "Help"="Returns the field state of the selected frame.\n\nAvailable Repeated Capabilities:\nSerialBus: SB1, SB2, SB3, SB4\r\n\nRemote-control command(s):\nBUS<m>:CAN:FRAMe<n>:CSSTate?"}, {"Level"=3, "Class Only"=FALSE, "Identifier"="RSSCOPE_ATTR_PROTOCOL_CAN_FRAME_ERROR_POSITION", "Descriptive Name"="Protocol CAN Frame Error Position", "Data Type"=1, "Command"="BUS{SerialBus}:CAN:FRAM<Frame>:BSEP?", "Access"=0, "Range Table"="", "Read Callback"="rsscope_FormatCANFrameRepCapReal64_ReadCallback.vi", "Write Callback"="", "Supported Models"="", "Instrument Options"="K3", "Flags"=0, "Help"="Queries the location of a bit stuffing error of the frame.\n\nAvailable Repeated Capabilities:\nSerialBus: SB1, SB2, SB3, SB4\r\n\nRemote-control command(s):\nBUS<m>:CAN:FRAMe<n>:BSEPosition?"}, {"Level"=3, "Class Only"=FALSE, "Identifier"="RSSCOPE_ATTR_PROTOCOL_CAN_FRAME_LABEL", "Descriptive Name"="Protocol CAN Frame Label", "Data Type"=2, "Command"="BUS{SerialBus}:CAN:FRAM<Frame>:SYMB?", "Access"=0, "Range Table"="", "Read Callback"="rsscope_FormatCANFrameRepCapString_ReadCallback.vi", "Write Callback"="", "Supported Models"="", "Instrument Options"="K3", "Flags"=0, "Help"="This attribute returns the symbolic label of the specified frame if the label list is enabled.\n\nAvailable Repeated Capabilities:\nSerialBus: SB1, SB2, SB3, SB4\r\n\nRemote-control command(s):\nBUS<m>:CAN:FRAMe<n>:SYMBol?"}, {"Level"=3, "Class Only"=FALSE, "Identifier"="RSSCOPE_ATTR_PROTOCOL_CAN_FRAME_NUMBER_OF_BYTES", "Descriptive Name"="Protocol CAN Frame Number Of Bytes", "Data Type"=0, "Command"="BUS{SerialBus}:CAN:FRAM<Frame>:NDBY?", "Access"=0, "Range Table"="", "Read Callback"="rsscope_FormatCANFrameRepCapInt32_ReadCallback.vi", "Write Callback"="", "Supported Models"="", "Instrument Options"="K3", "Flags"=0, "Help"="Returns the number of data bytes.\n\nAvailable Repeated Capabilities:\nSerialBus: SB1, SB2, SB3, SB4\r\n\nRemote-control command(s):\nBUS<m>:CAN:FRAMe<n>:NDBYtes?"}, {"Level"=3, "Class Only"=FALSE, "Identifier"="RSSCOPE_ATTR_PROTOCOL_CAN_FRAME_FORM_ERROR_CAUSE", "Descriptive Name"="Protocol CAN Frame Form Error Cause", "Data Type"=0, "Command"="BUS{SerialBus}:CAN:FRAM<Frame>:FERC?", "Access"=0, "Range Table"="RsScope_rngCANFrameFormErrorCause", "Read Callback"="rsscope_FormatCANFrameRepCapInt32_ReadCallback.vi", "Write Callback"="", "Supported Models"="", "Instrument Options"="K3", "Flags"=0, "Help"="Returns information on a form error, if the frame status query returned a FORM error.\n\nAvailable Repeated Capabilities:\nSerialBus: SB1, SB2, SB3, SB4\r\n\nRemote-control command(s):\nBUS<m>:CAN:FRAMe<n>:FERCause?"}, {"Level"=3, "Class Only"=FALSE, "Identifier"="RSSCOPE_ATTR_PROTOCOL_CAN_FD_FRAME_STUFF_COUNT", "Descriptive Name"="Protocol CAN FD Frame Stuff Count", "Data Type"=0, "Command"="BUS{SerialBus}:CAN:FDAT:FRAM<Frame>:SCV?", "Access"=0, "Range Table"="", "Read Callback"="rsscope_FormatCANFrameRepCapInt32_ReadCallback.vi", "Write Callback"="", "Supported Models"="", "Instrument Options"="K3", "Flags"=0, "Help"="Returns the stuff bit count modulo 8 value.\n\nAvailable Repeated Capabilities:\nSerialBus: SB1, SB2, SB3, SB4\r\n\nRemote-control command(s):\nBUS<m>:CAN:FDATa:FRAMe<n>:SCValue?"}, {"Level"=3, "Class Only"=FALSE, "Identifier"="RSSCOPE_ATTR_PROTOCOL_CAN_SELECTED_BYTE", "Descriptive Name"="Protocol CAN Selected Byte", "Data Type"=0, "Command"="", "Access"=2, "Range Table"="", "Read Callback"="", "Write Callback"="", "Supported Models"="", "Instrument Options"="", "Flags"=0, "Help"="Sets selector repeated capability Byte.\n\nAvailable Repeated Capabilities:\nNone\n\nRemote-control command(s):\ncmd"}, {"Level"=3, "Class Only"=FALSE, "Identifier"="RSSCOPE_ATTR_PROTOCOL_CAN_FRAME_BYTE_DATA", "Descriptive Name"="Protocol CAN Frame Byte Data", "Data Type"=0, "Command"="BUS{SerialBus}:CAN:FRAM<Frame>:BYTE<Byte>:VAL?", "Access"=0, "Range Table"="", "Read Callback"="rsscope_FormatCANByteRepCapInt32_ReadCallback.vi", "Write Callback"="", "Supported Models"="", "Instrument Options"="K3", "Flags"=0, "Help"="Value of the specified byte.\n\nAvailable Repeated Capabilities:\nSerialBus: SB1, SB2, SB3, SB4\r\n\nRemote-control command(s):\nBUS<m>:CAN:FRAMe<n>:BYTE<o>:VALue?"}, {"Level"=3, "Class Only"=FALSE, "Identifier"="RSSCOPE_ATTR_PROTOCOL_CAN_FRAME_BYTE_STATUS", "Descriptive Name"="Protocol CAN Frame Byte Status", "Data Type"=0, "Command"="BUS{SerialBus}:CAN:FRAM<Frame>:BYTE<Byte>:STAT?", "Access"=0, "Range Table"="RsScope_rngCANFrameMessageStatus", "Read Callback"="rsscope_FormatCANByteRepCapInt32_ReadCallback.vi", "Write Callback"="", "Supported Models"="", "Instrument Options"="K3", "Flags"=0, "Help"="Returns the data state for the specified frame.\n\nAvailable Repeated Capabilities:\nSerialBus: SB1, SB2, SB3, SB4\r\n\nRemote-control command(s):\nBUS<m>:CAN:FRAMe<n>:BYTE<o>:STATe?"}, {"Level"=3, "Class Only"=TRUE, "Identifier"="", "Descriptive Name"="Time Segment", "Data Type"=0, "Command"="", "Access"=0, "Range Table"="", "Read Callback"="", "Write Callback"="", "Supported Models"="", "Instrument Options"="", "Flags"=0, "Help"="Selects Time Segment"}, {"Level"=4, "Class Only"=FALSE, "Identifier"="RSSCOPE_ATTR_PROTOCOL_CAN_SAMPLE_POINT_ABS", "Descriptive Name"="Protocol CAN Sample Point Abs", "Data Type"=0, "Command"="BUS{SerialBus}:CAN:T{CANTimeSeg}S", "Access"=2, "Range Table"="RsScope_rngProtocolCANSamplePointAbs", "Read Callback"="", "Write Callback"="", "Supported Models"="", "Instrument Options"="K0|K3", "Flags"=0, "Help"="Set the number of time quanta before the sample point (T1Segment) and after the sample point (T2Segment). T1Segment comprises the segments Synch_seg, Prop_seg, and Phase_seg1 which are specified in the CAN standard. T2Segment
